vi "Create Timer.vi"(4 "error in (no error)":errorcluster, 5 "return exisiting (F)":bool, 6 "Timer Accuracy":enum16{"1 ms", "10 ms"}(ring), 7 "name (unnamed)":string) -> (0 "error out":errorcluster, 1 "created new":bool, 3 "timer":T1)   [LabVIEW 2011]
doc: "Looks up an existing timer or creates a new timer and returns a refnum that you can use when calling other timer VIs.\n\n© Copyright 1999\nCal-Bay Systems, Inc.\nwritten by James Kring"
uses:
  Timer Refnum.ctl
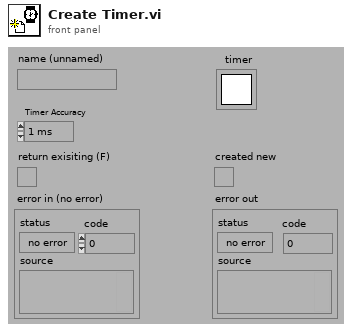
[diagram p1: front panel]
types:
  T1 = typedef "Timer Refnum.ctl" = refnum<k1>
  T2 = enum16{"open ref", "lookup ref", "close ref", "test ref", "start", "stop", "wait", "reset", "increment # waiting", "decrement #waiting"}
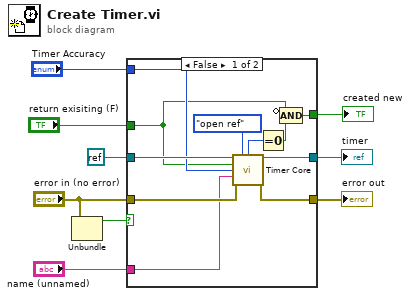
[diagram p0: block diagram]
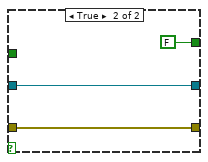
[diagram p2: hidden frame]
diagram:
  n1 = Unbundle("error in (no error)") -> ("status"=w8:bool)  [unwired: 2 out]
  n2 = case shown="False" w8 {
    tunnel: [w20 w22] -> w7
    tunnel: "error in (no error)" -> [w19 w23]
    tunnel: [w18 w23] -> w6
    tunnel: refnum<k0> refnum -> [w16 w22]
    tunnel: "name (unnamed)" -> [w17 _]
    tunnel: "return exisiting (F)" -> [w10 _]
    tunnel: [w11 FALSE] -> w2
    tunnel: "Timer Accuracy" -> [w14 _]
    frame False {
      n3 = call "Timer Core.vi"("timer"=w16, "function"=T2."open ref", "return exisiting (F)"=w10, "Accuracy"=w14, "name"=w17, "error in (no error)"=w19) -> ("error"=w15:i32, "timer out"=w20:T1, "error out"=w18:errorcluster)  [unwired: 3 in, 4 out]
      n4 = Equal To 0?(x=w15) -> (x = 0?=w12:bool)
      n5 = Compound Arithmetic op=AND(invert w10, w12) -> (w11:bool)
    }
    frame True {
    }
  }
  "error out" <- w6
  "timer" <- w7
  "created new" <- w2
